vi "Result.Numeric Value Fix for NaN.vi"(11 "Numeric":dbl) -> (3 "Numeric Out":dbl)   [LabVIEW 2018]
panel:
  out "Str":string
  out "-Inf":bool
  out "+Inf":bool
  out "NaN":bool
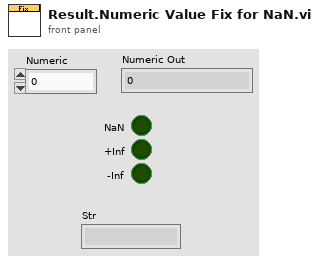
[diagram p1: front panel]
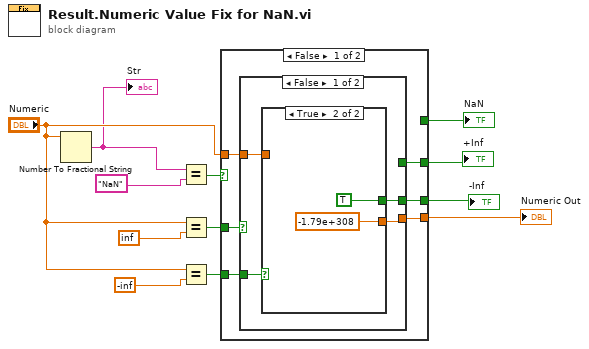
[diagram p0: block diagram]
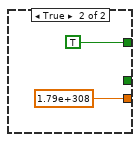
[diagram p3: hidden frame]
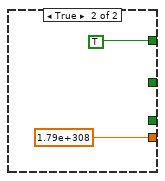
[diagram p4: hidden frame]
diagram:
  n1 = Number To Fractional String(number="Numeric") -> (F-format string=w1:string)  [unwired: 3 in]
  "Str" <- w1
  n2 = Equal?(x=w1, y="NaN") -> (x = y?=w10:bool)
  n3 = Equal?(x="Numeric", y=inf) -> (x = y?=w8:bool)
  n4 = Equal?(x="Numeric", y=-inf) -> (x = y?=w7:bool)
  n5 = case shown="False" w10 {
    tunnel: [w17 1.79e+308] -> w9
    tunnel: w8 -> [w18 _]
    tunnel: w7 -> [w16 _]
    tunnel: "Numeric" -> [w15 _]
    tunnel: [_ TRUE] -> w6
    tunnel: [w14 _] -> w5
    tunnel: [w13 _] -> w4
    frame False {
      n6 = case shown="False" w18 {
        tunnel: [w21 1.79e+308] -> w17
        tunnel: w16 -> [w22 _]
        tunnel: w15 -> [w20 _]
        tunnel: [_ TRUE] -> w14
        tunnel: [w19 _] -> w13
        frame False {
          n7 = case shown="True" w22 {
            tunnel: [w23 -1.79e+308] -> w21
            tunnel: w20 -> [w23 _]
            tunnel: [_ TRUE] -> w19
            frame False {
            }
            frame True {
            }
          }
        }
        frame True {
        }
      }
    }
    frame True {
    }
  }
  "Numeric Out" <- w9
  "NaN" <- w6
  "+Inf" <- w5
  "-Inf" <- w4
